vi "PH_Beckhoff_PP_Control.declare digital InputTags.vi"() -> (0 "Digital Inputs":T2, 1 "Description":string)   [LabVIEW 2014, in "PH_Beckhoff_PP_Control.lvlib"]
uses:
  PH_Beckhoff_PP_Control.lvlib
  PH_Beckhoff/PH_Beckhoff.Digital Inputs.ctl
  PH_Beckhoff_PP_Control.PP Conductivity Tags.ctl
  PH_Beckhoff_PP_Control.PP Mercury Tags.ctl
  PH_Beckhoff/PH_Beckhoff.lvlib
panel:
  in  "Digital Input Value":T1
  out "Right Size?":bool
  # "Let this VI run to check the size!"
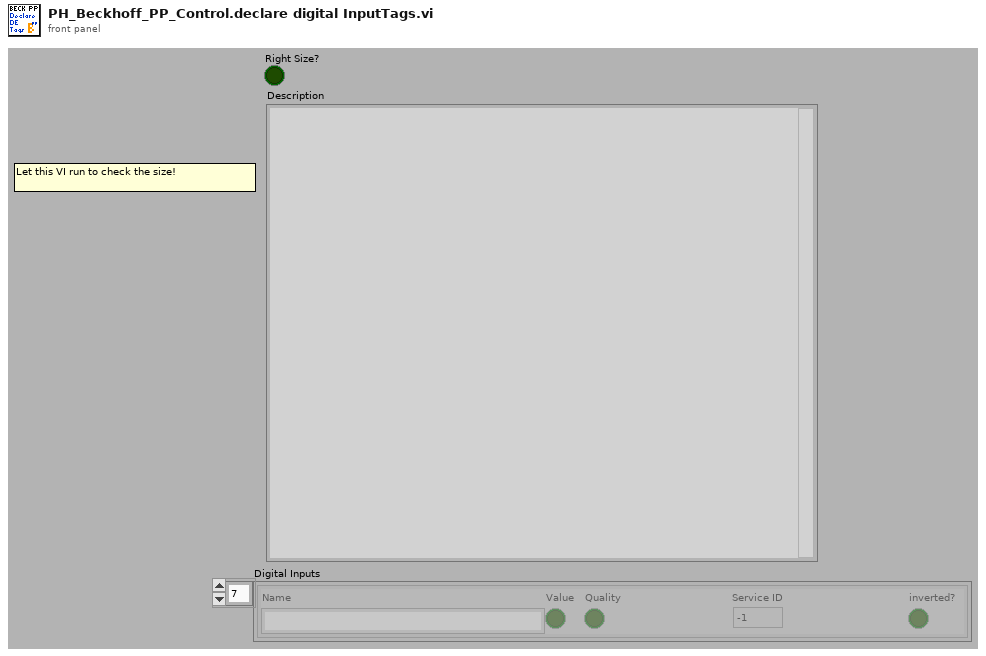
[diagram p1: front panel]
types:
  T1 = cluster{"Name":string, "Value":bool, "Quality":bool, "Service ID":i32, "inverted?":bool}
  T2 = typedef "PH_Beckhoff.lvlib/PH_Beckhoff.Digital Inputs.ctl" = cluster{"Name":string, "Value":bool, "Quality":bool, "Service ID":i32, "inverted?":bool}[]
  T3 = typedef "PH_Beckhoff_PP_Control.lvlib/PH_Beckhoff_PP_Control.PP Mercury Tags.ctl" = enum16{"Device-on", "Alarm", "on-since", "Concentration", "Status"}
  T4 = typedef "PH_Beckhoff_PP_Control.lvlib/PH_Beckhoff_PP_Control.PP Conductivity Tags.ctl" = enum16{"Device-on", "Conductivity-2-high", "Temperature-not-2-low", "Alarm", "Conductivity", "Status"}
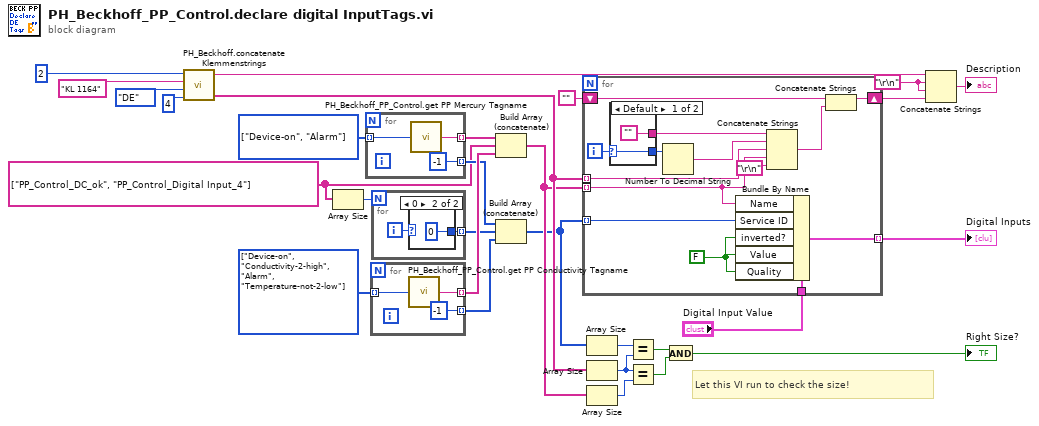
[diagram p0: block diagram]
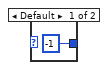
[diagram p2: hidden frame]
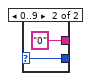
[diagram p3: hidden frame]
diagram:
  w5 = T3[] [enum."Device-on", enum."Alarm"] items=["Device-on", "Alarm", "on-since", "Concentration", "Status"]
  w16 = T4[] [enum."Device-on", enum."Conductivity-2-high", enum."Alarm", enum."Temperature-not-2-low"] items=["Device-on", "Conductivity-2-high", "Temperature-not-2-low", "Alarm", "Conductivity", "Status"]
  w1 = string[] ["PP_Control_DC_ok", "PP_Control_Digital Input_4"]
  w27 = "\r\n"
  # "Let this VI run to check the size!"
  n1 = call "PH_Beckhoff.concatenate Klemmenstrings.vi"("# of In- or Outputs"=4, "Type"=enum16{"AE", "AA", "DE", "DA"}."DE", "Klemmenname"="KL 1164", "Quantity"=2) -> ("concatenated string array"=w20:string[], "\"<Type>: <Quantity> x <Klemmenname>\""=w21:string)  [unwired: 1 out]
  n2 = Array Size(array=w1) -> (size(s)=w2:i32)
  n3 = for {
    tunnel: w5 -> [w32] mode=indexing
    tunnel: [w31] -> w4 mode=indexing
    tunnel: [-1] -> w3 mode=indexing
    n4 = call "PH_Beckhoff_PP_Control.get PP Mercury Tagname.vi"("PP Mercury Tag"=w32) -> ("PP Mercury Tagname"=w31:string)
  }
  n5 = for {
    tunnel: [w35] -> w15 mode=indexing
    tunnel: [-1] -> w14 mode=indexing
    tunnel: w16 -> [w33] mode=indexing
    n6 = call "PH_Beckhoff_PP_Control.get PP Conductivity Tagname.vi"("PP Conductivity Tag"=w33) -> ("PP Conductivity Tagname"=w35:string)
  }
  n7 = for {
    N: w2 -> [_]
    tunnel: [w37] -> w13 mode=indexing
    i -> [w36]
    n8 = case shown="0" w36 {
      tunnel: [-1 0] -> w37
      frame Default {
      }
      frame 0 {
      }
    }
  }
  n9 = Build Array (concatenate)(w4, w1, w15) -> (w12:string[])
  n10 = Build Array (concatenate)(w3, w13, w14) -> (w11:i32[])
  n11 = for {
    tunnel: w12 -> [w44] mode=indexing
    tunnel: w20 -> [w49] mode=indexing
    shift-right: [w47] -> w28
    shift-left: "" -> [w46]
    tunnel: "Digital Input Value" -> [w45]
    tunnel: [w43] -> w17 mode=indexing
    tunnel: w11 -> [w40] mode=indexing
    i -> [w53]
    w42 = FALSE ("Quality")
    n12 = case shown="Default" w53 {
      selector: w53 -> [w54 w57]
      tunnel: [w54 w57] -> w52
      tunnel: ["" "0"] -> w51
      frame Default {
      }
      frame 0..9 {
      }
    }
    n13 = Number To Decimal String(number=w52) -> (decimal integer string=w50:string)  [unwired: 1 in]
    n14 = Bundle By Name(cluster=w45, "Name"=w44, "Service ID"=w40, "inverted?"=w42, "Value"=w42, "Quality"=w42) -> (w43:T1)
    n15 = Concatenate Strings(w51, w50, w49, w44, "\r\n") -> (w48:string)
    n16 = Concatenate Strings(w46, w48) -> (w47:string)
  }
  "Digital Inputs" <- w17
  n17 = Array Size(array=w11) -> (size(s)=w10:i32)
  n18 = Array Size(array=w20) -> (size(s)=w9:i32)
  n19 = Array Size(array=w12) -> (size(s)=w19:i32)
  n20 = Equal?(x=w10, y=w9) -> (x = y?=w8:bool)
  n21 = Equal?(x=w9, y=w19) -> (x = y?=w7:bool)
  n22 = And(x=w8, y=w7) -> (x .and. y?=→"Right Size?":bool)
  n23 = Concatenate Strings(w21, w27, w27, w28) -> (→"Description":string)
